vi "23 Input Scaling (2017).vi"(1 "Input (Raw)":dynamicdata(waveform)) -> (0 "Output (Scaled)":dynamicdata(waveform))   [LabVIEW 2017]
uses:
  24 Global Front Panel (2017).vi
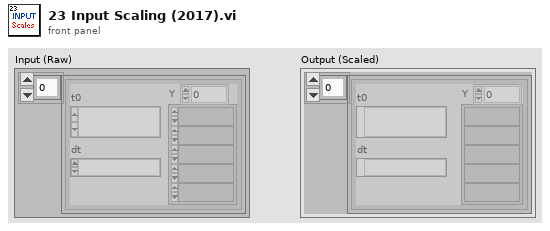
[diagram p1: front panel]
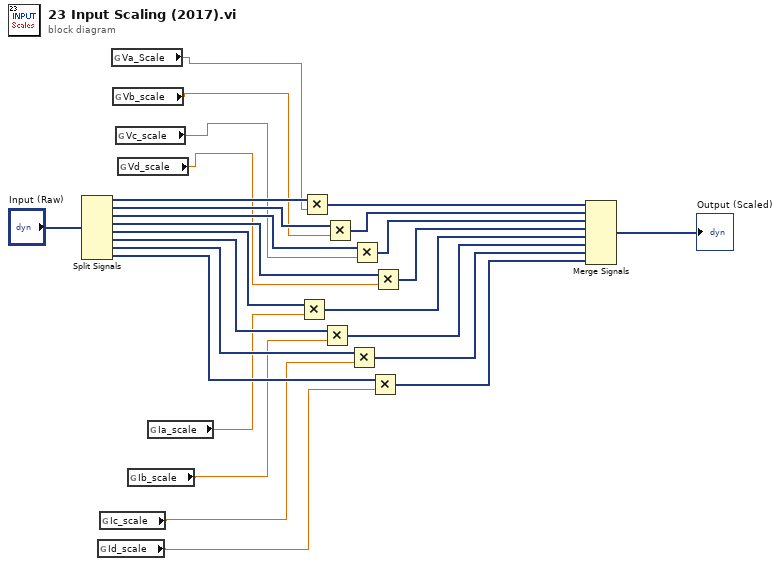
[diagram p0: block diagram]
diagram:
  n1 = Split Signals("Input (Raw)") -> (w24:dynamicdata, w22:dynamicdata, w20:dynamicdata, w18:dynamicdata, w16:dynamicdata, w15:dynamicdata, w14:dynamicdata, w10:dynamicdata)  [unwired: 8 in]
  n2 = global read "24 Global Front Panel (2017).vi" "Id_scale"() -> (w4:dbl)
  n3 = global read "24 Global Front Panel (2017).vi" "Ic_scale"() -> (w5:dbl)
  n4 = global read "24 Global Front Panel (2017).vi" "Va_Scale"() -> (w8:dbl)
  n5 = global read "24 Global Front Panel (2017).vi" "Vb_scale"() -> (w3:dbl)
  n6 = global read "24 Global Front Panel (2017).vi" "Vc_scale"() -> (w2:dbl)
  n7 = global read "24 Global Front Panel (2017).vi" "Vd_scale"() -> (w1:dbl)
  n8 = global read "24 Global Front Panel (2017).vi" "Ib_scale"() -> (w6:dbl)
  n9 = global read "24 Global Front Panel (2017).vi" "Ia_scale"() -> (w7:dbl)
  n10 = Multiply(x=w16, y=w7) -> (x*y=w13:dynamicdata)
  n11 = Multiply(x=w24, y=w8) -> (x*y=w25:dynamicdata)
  n12 = Multiply(x=w15, y=w6) -> (x*y=w12:dynamicdata)
  n13 = Multiply(x=w22, y=w3) -> (x*y=w21:dynamicdata)
  n14 = Multiply(x=w14, y=w5) -> (x*y=w11:dynamicdata)
  n15 = Multiply(x=w20, y=w2) -> (x*y=w19:dynamicdata)
  n16 = Multiply(x=w10, y=w4) -> (x*y=w9:dynamicdata)
  n17 = Multiply(x=w18, y=w1) -> (x*y=w17:dynamicdata)
  n18 = Merge Signals(w25, w21, w19, w17, w13, w12, w11, w9) -> (→"Output (Scaled)":dynamicdata)
